vi "Multimeter.vi"() -> ()   [LabVIEW 2020]
panel:
  out "Current  (mA)":dbl
  in  "Voltage\n\n\n\n\nCurrent":bool
  in  "Reset Real-Time Graph":bool
  out "Real-Time Graph":cluster{"Y":dbl[], "Y":dbl[]}[](graph)
  in  "Start Collecting Data":bool
  out "Voltage (mV)":dbl
  in  "Min Value":dbl=-5.0
  in  "Max Value":dbl=5.0
  in  "Analog Input Channel":refnum<k21>
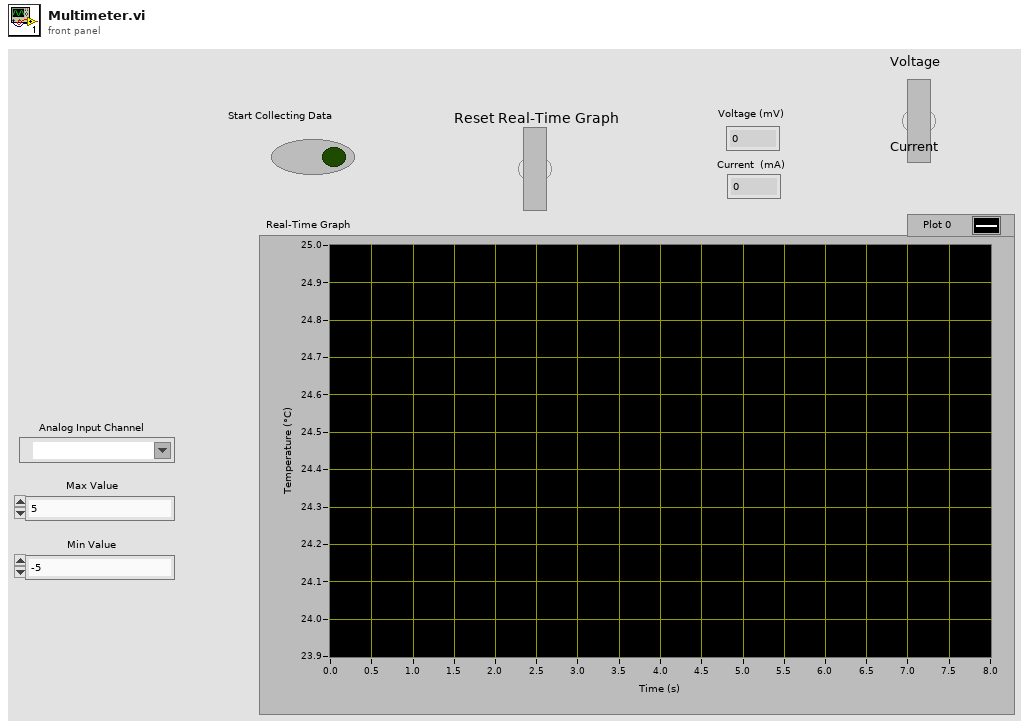
[diagram p1: front panel]
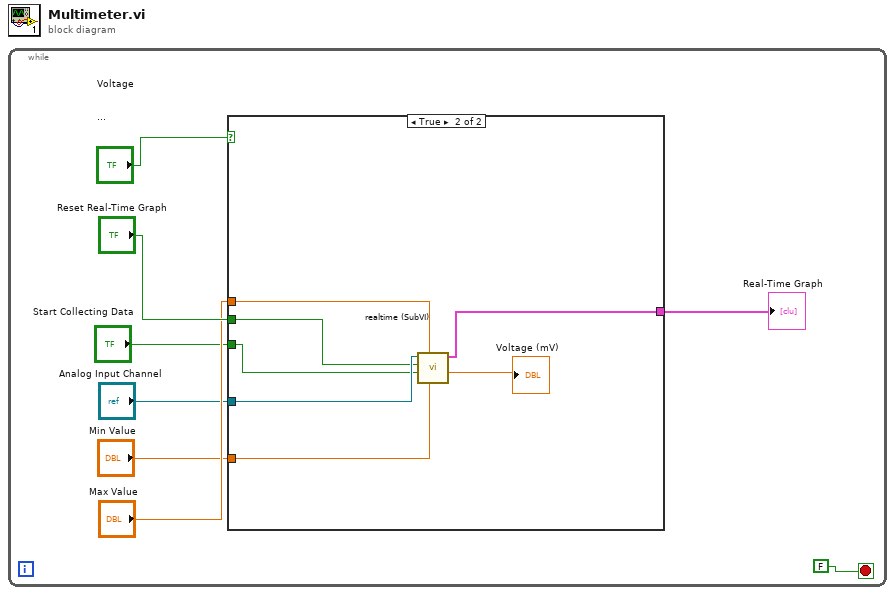
[diagram p0: block diagram]
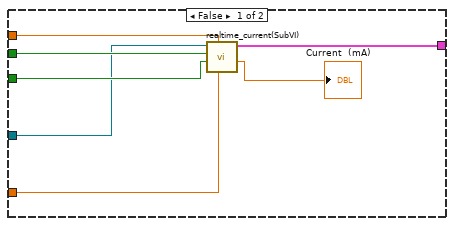
[diagram p2: hidden frame]
diagram:
  n1 = while {
    stop <- FALSE stop-if-true
    n2 = case shown="True" "Voltage\n\n\n\n\nCurrent" {
      tunnel: [w14 w16] -> w7
      tunnel: "Reset Real-Time Graph" -> [w13 w19]
      tunnel: "Max Value" -> [w12 w22]
      tunnel: "Start Collecting Data" -> [w11 w20]
      tunnel: "Min Value" -> [w10 w18]
      tunnel: "Analog Input Channel" -> [w9 w21]
      frame False {
        n3 = call "realtime_current(SubVI) .vi"("Min Value"=w10, "Max Value"=w12, "Start Collecting Real-Time Data"=w11, "Reset Real-Time Graph"=w13, "Refnum in"=w9) -> ("Current (mA)"=→"Current  (mA)":dbl, "XY Graph"=w14:cluster{"X":dbl[], "Y":dbl[]}[])  [unwired: 4 in, 1 out]
      }
      frame True {
        n4 = call "realtime (SubVI).vi"("Min Value"=w18, "Max Value"=w22, "Start Collecting Real-Time Data"=w20, "Reset Real-Time Graph"=w19, "Refnum in"=w21) -> ("Current Voltage (mV)"=→"Voltage (mV)":dbl, "XY Graph"=w16:cluster{"X":dbl[], "Y":dbl[]}[])  [unwired: 4 in, 1 out]
      }
    }
    "Real-Time Graph" <- w7
  }
